vi "Handle Failure Action Change Event.vi"(7 "Assert Data":T1, 8 "error in (no error)":errorcluster, 10 "Created New?":bool, 11 "Failure Action References":T2) -> (0 "error out":errorcluster)   [LabVIEW 2016, in "AssertEngine.lvlib"]
uses:
  AssertEngine.lvlib
  Failure Action References.ctl
  Log Assert/Assert Data.ctl
  Failure Action.lvclass
  Abort Application/Abort Application.lvclass
  D:/Work/Projects/Actor_Assert_API/Core/AssertEngine/Failure Actions/Failure Action.lvclass
  Log To File/Log To File.lvclass
  Pause Execution/Pause Execution.lvclass
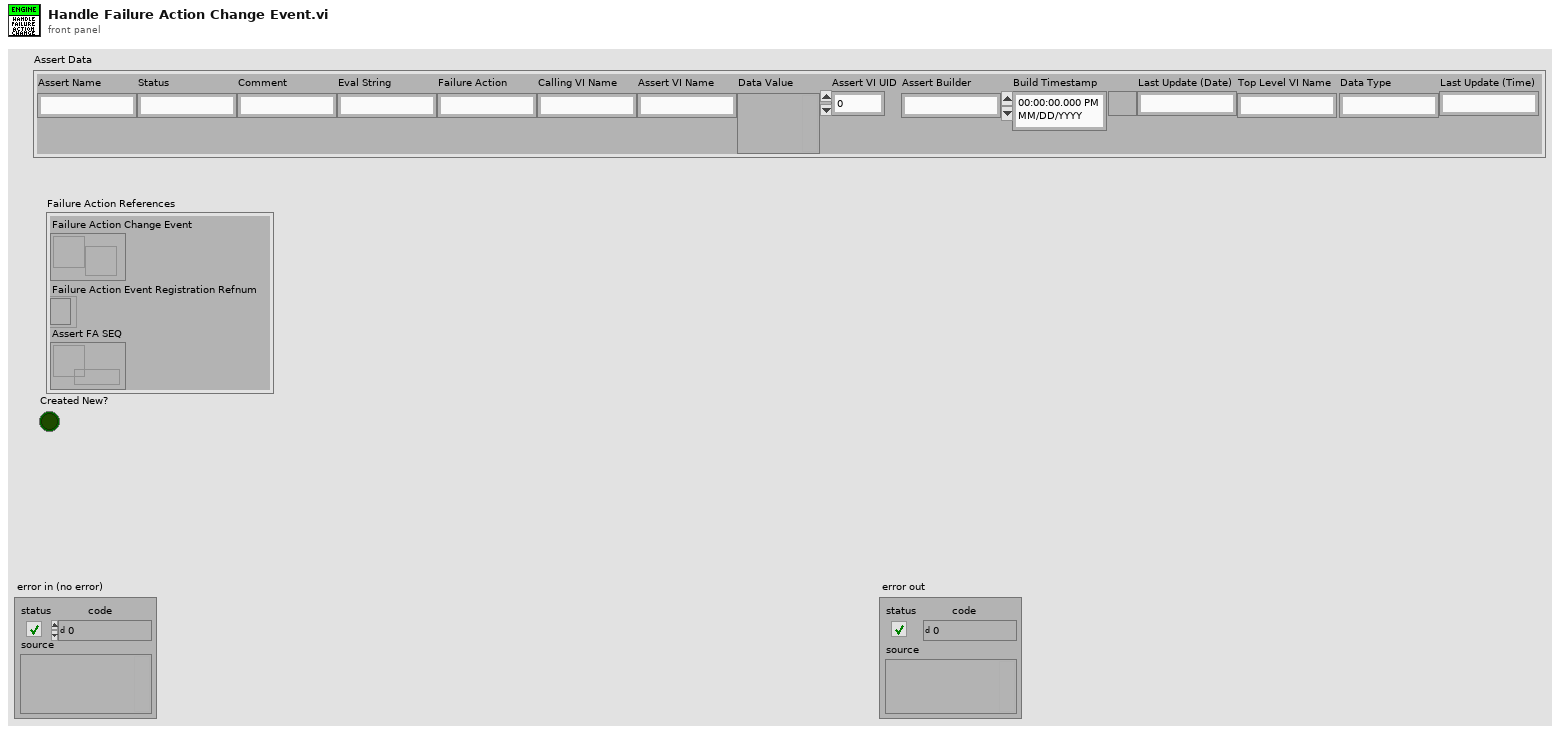
[diagram p1: front panel]
types:
  T1 = typedef "AssertEngine.lvlib/Assert Data.ctl" = cluster{"Assert Name":string, "Status":string, "Comment":string, "Eval String":string, "Failure Action":string, "Calling VI Name":string, "Assert VI Name":string, "Data Value":variant, "Assert VI UID":i32, "Assert Builder":string, "Build Timestamp":timestamp, "Last Update (Date)":string, "Top Level VI Name":string, "Data Type":string, "Last Update (Time)":string}
  T2 = typedef "AssertEngine.lvlib/Failure Action References.ctl" = cluster{"Failure Action Change Event":refnum<user-event>, "Failure Action Event Registration Refnum":refnum<event-registration>, "Assert FA SEQ":refnum<queue>}
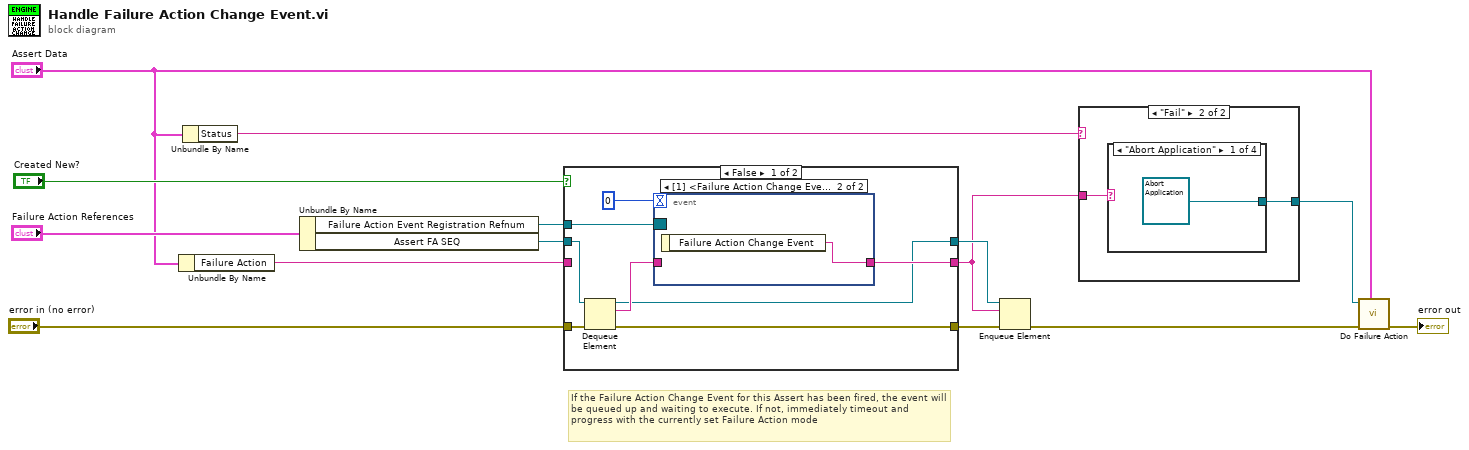
[diagram p0: block diagram]
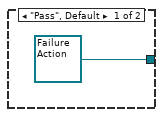
[diagram p2: hidden frame]
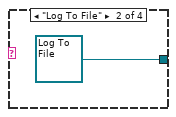
[diagram p3: hidden frame]
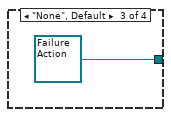
[diagram p4: hidden frame]
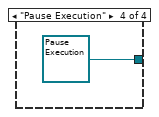
[diagram p5: hidden frame]
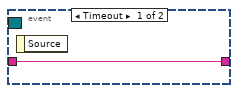
[diagram p6: hidden frame]
diagram:
  # "If the Failure Action Change Event for this Assert has been fired, the event will be queued up and waiting to execute. If not, immediately timeout and progress with the currently set Failure Action mode"
  n1 = Unbundle By Name("Assert Data") -> ("Failure Action"=w10:string)
  n2 = Unbundle By Name("Assert Data") -> ("Status"=w6:string)
  n3 = Unbundle By Name("Failure Action References") -> ("Failure Action Event Registration Refnum"=w11:refnum<event-registration>, "Assert FA SEQ"=w14:refnum<queue>)
  n4 = case shown="False" "Created New?" {
    tunnel: [w20 w25] -> w5
    tunnel: w11 -> [w21 _]
    tunnel: w14 -> [w19 w26]
    tunnel: "error in (no error)" -> [w17 w27]
    tunnel: [w16 w27] -> w13
    tunnel: [w15 w26] -> w12
    tunnel: w10 -> [_ w25]
    frame False {
      n5 = Dequeue Element(queue=w19, error in (no error)=w17) -> (queue out=w15:refnum<queue>, element=w18:string, error out=w16:errorcluster)  [unwired: 1 in, 1 out]
      n6 = event shown="[1] <Failure Action Change Event>: User Event" {
        selector: w21 -> [_ _]
        dyn-events: _ -> [_ _]
        timeout: 0 -> [_ _]
        tunnel: [w23 w24] -> w20
        tunnel: w18 -> [w23 _]
        event Timeout {
          n7 = event-data() -> ()  [unwired: 1 in, 1 out]
        }
        event User Event {
          n8 = event-data() -> ("Failure Action Change Event"=w24:string)  [unwired: 1 in]
        }
      }
    }
    frame True {
      # "Takes the default failure action on the first call but thereafter looks in the SEQ"
    }
  }
  n9 = Enqueue Element(queue=w12, element=w5, error in (no error)=w13) -> (error out=w4:errorcluster)  [unwired: 1 in, 2 out]
  n10 = case shown="\"Fail\"" w6 {
    tunnel: w5 -> [_ w30]
    tunnel: [refnum<class "Failure Action.lvclass"> refnum ("AssertEngine.lvlib:Failure Action.lvclass") w29] -> w2
    frame "Pass", Default {
    }
    frame "Fail" {
      n11 = case shown="\"Abort Application\"" w30 {
        tunnel: [refnum<class "Abort Application.lvclass"> refnum ("AssertEngine.lvlib:Abort Application.lvclass") refnum<class "Log To File.lvclass"> refnum ("AssertEngine.lvlib:Log To File.lvclass") refnum<class "Failure Action.lvclass"> refnum ("AssertEngine.lvlib:Failure Action.lvclass") refnum<class "Pause Execution.lvclass"> refnum ("AssertEngine.lvlib:Pause Execution.lvclass")] -> w29
        frame "Abort Application" {
        }
        frame "Log To File" {
        }
        frame "None", Default {
        }
        frame "Pause Execution" {
        }
      }
    }
  }
  n12 = call-dynamic "Do Failure Action.vi"("Assert Data"="Assert Data", "error in (no error)"=w4, "Failure Action in"=w2) -> ("error out"=→"error out":errorcluster)  [unwired: 8 in]
